vi "建立数组函数.vi"() -> ()   [LabVIEW 2010]
panel:
  out "两个数值\n建成一维数组":i32[](array[numeric])
  out "单个数值\n建成一个数组":i32[](array[numeric])
  out "两个一维数组\n连接在一起":i32[](array[numeric])
  out "两个一维数组\n建成二维数组":i32[][](array[numeric])
  out "新建的数组":string[][](array[string])
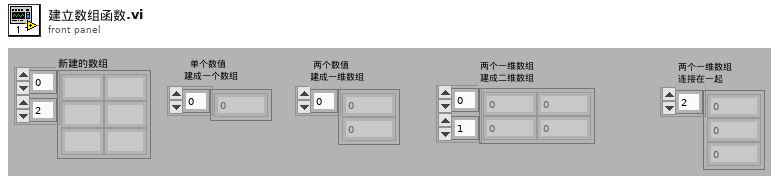
[diagram p1: front panel]
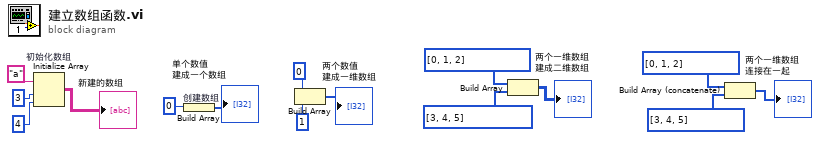
[diagram p0: block diagram]
diagram:
  n1 = Initialize Array "初始化数组"("a", 3 ("dimension size"), 4 ("dimension size")) -> (→"新建的数组":string[][])
  n2 = Build Array "创建数组"(0) -> (→"单个数值\n建成一个数组":i32[])
  n3 = Build Array(0, 1) -> (→"两个数值\n建成一维数组":i32[])
  n4 = Build Array(i32[] [0, 1, 2], i32[] [3, 4, 5]) -> (→"两个一维数组\n建成二维数组":i32[][])
  n5 = Build Array (concatenate)(i32[] [0, 1, 2], i32[] [3, 4, 5]) -> (→"两个一维数组\n连接在一起":i32[])
